vi "Specific Error Handler(RT).vi"   [LabVIEW 2014]
doc: "Checks an error against a set of error handling instructions configured by the express VI.\n\nIf the error to check is in the list of errors to handle, the VI extracts the error handling information and performs the apropriate actions.\n\nThis VI will never detect an error with a code of 0, even if the status is set to true.\n\nThis VI is optimized for Real-Time applications. An alternate version for Windows VIs exists."
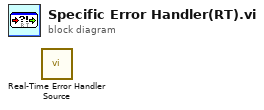
[diagram p0: block diagram]
diagram:
  n1 = call "Real-Time Error Handler Source"() -> ()  [unwired: 12 in, 4 out]
